vi "Write into Array of Instrument addresses.vi"(8 "error in (no error)":errorcluster, 10 "new element/subarray":refnum<class "Message Enqueuer.lvclass">, 11 "Instrument Finder in":refnum<class "Instrument Finder.lvclass">) -> (0 "error out":errorcluster, 3 "Instrument Finder out":refnum<class "Instrument Finder.lvclass">)   [LabVIEW 2016, in "SetUp VIs.lvlib" / "Instrument Finder.lvclass"]
uses:
  Instrument Finder.lvclass
  <vilib>/ActorFramework/Message Enqueuer/Message Enqueuer.lvclass
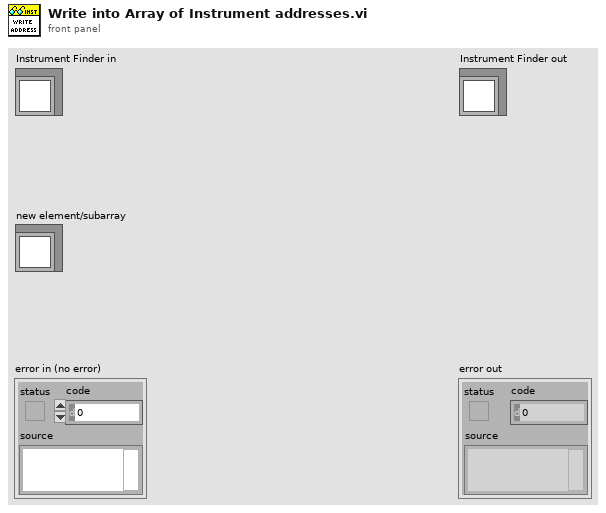
[diagram p1: front panel]
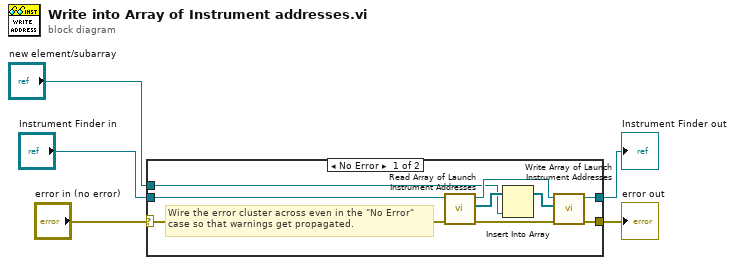
[diagram p0: block diagram]
diagram:
  n1 = case shown="No Error" "error in (no error)" {
    selector: "error in (no error)" -> [w8 w16]
    tunnel: [w6 w16] -> w4
    tunnel: [w12 w15] -> w2
    tunnel: "Instrument Finder in" -> [w14 w15]
    tunnel: "new element/subarray" -> [w9 _]
    frame No Error {
      # "Wire the error cluster across even in the \"No Error\"\ncase so that warnings get propagated."
      n2 = call-dynamic "Read Array of Launch Instrument Addresses.vi"("error in (no error)"=w8, "Instrument Finder in"=w14) -> ("error out"=w7:errorcluster, "Array of Launch Instrument Addresses"=w11:refnum<class "Message Enqueuer.lvclass">[], "Instrument Finder out"=w13:refnum<class "Instrument Finder.lvclass">)  [unwired: 7 in]
      n3 = Insert Into Array(array=w11, new element=w9) -> (w10:refnum<class "Message Enqueuer.lvclass">[])  [unwired: 1 in]
      n4 = call-dynamic "Write Array of Launch Instrument Addresses.vi"("error in (no error)"=w7, "Array of Launch Instrument Addresses"=w10, "Instrument Finder in"=w13) -> ("error out"=w6:errorcluster, "Instrument Finder out"=w12:refnum<class "Instrument Finder.lvclass">)  [unwired: 7 in]
    }
    frame Error {
    }
  }
  "error out" <- w4
  "Instrument Finder out" <- w2
